vi "Close_Baxter.vi"(0 "error in":errorcluster, 3 "node":string) -> (1 "error out":errorcluster)   [LabVIEW 2015]
doc: "This will close all topics and disable Baxter."
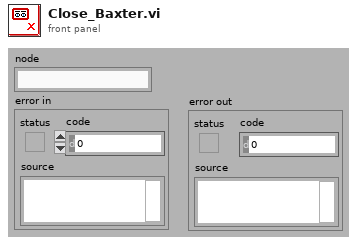
[diagram p1: front panel]
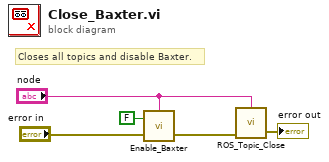
[diagram p0: block diagram]
diagram:
  # "Closes all topics and disable Baxter."
  n1 = call "Enable_Baxter.vi"("error in"="error in", "Enable?"=FALSE, "node"="node") -> ("error out"=w3:errorcluster)  [unwired: 1 in]
  n2 = call "ROS_Topic_Close.vi"("error in"=w3, "node"="node") -> ("error out"=→"error out":errorcluster)  [unwired: 2 in]
